vi "俄罗斯方块-是否可操作.vi"(8 "Y":i8, 9 "X":i8, 10 "形状数组":u32[][](array[colorbox]), 11 "主窗数组":u32[][](array[colorbox])) -> (3 "是否可操作":bool=TRUE)   [LabVIEW 2016]
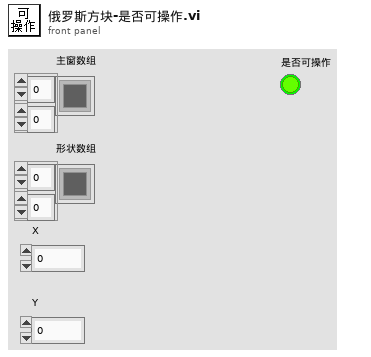
[diagram p1: front panel]
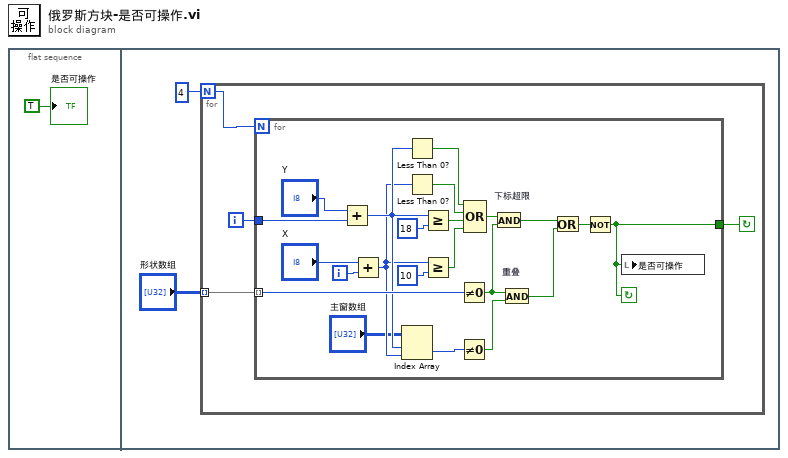
[diagram p0: block diagram]
diagram:
  n1 = flat-sequence {
    frame #0 {
      "是否可操作" <- TRUE
    }
    frame #1 {
      n2 = for {
        N: 4 -> [w7]
        tunnel: "形状数组" -> [w6] mode=indexing
        i -> [w5]
        stop <- w4 continue-if-true
        n3 = for {
          N: w7 -> [_]
          tunnel: w6 -> [w26] mode=indexing
          tunnel: w5 -> [w29]
          tunnel: [w8] -> w4
          i -> [w28]
          stop <- w8 continue-if-true
          n4 = Add(x="Y", y=w29) -> (x+y=w17:i32)
          n5 = Add(x="X", y=w28) -> (x+y=w15:i32)
          n6 = Index Array(array="主窗数组", index (row)=w17, index (col)=w15) -> (element=w27:u32)
          n7 = Less Than 0?(x=w17) -> (x < 0?=w21:bool)
          n8 = Less Than 0?(x=w15) -> (x < 0?=w20:bool)
          n9 = Greater Or Equal?(x=w17, y=18) -> (x >= y?=w19:bool)
          n10 = Greater Or Equal?(x=w15, y=10) -> (x >= y?=w18:bool)
          n11 = Not Equal To 0?(x=w26) -> (x != 0?=w13:bool)
          n12 = Not Equal To 0?(x=w27) -> (x != 0?=w12:bool)
          n13 = Compound Arithmetic op=OR ("复合运算")(w21, w20, w19, w18) -> (w25:bool)
          n14 = And "下标超限"(x=w25, y=w13) -> (x .and. y?=w24:bool)
          n15 = And "重叠"(x=w13, y=w12) -> (x .and. y?=w23:bool)
          n16 = Or(x=w24, y=w23) -> (x .or. y?=w22:bool)
          n17 = Not(x=w22) -> (.not. x?=w8:bool)
          n18 = local write "是否可操作"(w8) -> ()
        }
      }
    }
  }
